vi "CRYO_DAQ_LSI218.vi"() -> ()   [LabVIEW 2017]
uses:
  USBData.lvclass
panel:
  in  "Stop Button":bool
  out "Cycle #":u32=16
  out "Time of Last Measurement":timestamp=timestamp(3679551576.02604 s since 1904-01-01)
  in  "wait (ms)":u32=1000
  in  "?":enum32{"CONFIG", "MEASUREMENT"}(tab)
  in  "USBSettings":T1(array[cluster])=[{"Label"="GXS450", "FileFormat"="%2.2f", "Physical CH"="Dev2/ai0", "ConversionType"={"Type"=enum."CC-10_LOG", "ConversionParameters"=[0.5, 9.0, 0.0, 1.0]}, "VoltageLimits"=[0.0, 10.0]}, {"Label"="Vacuum insluation", "FileFormat"="%2.2f", "Physical CH"="Dev2/ai1", "ConversionType"={"Type"=enum."CC-10_LOG", "ConversionParameters"=[0.5, 9.0, 0.0, 1.0]}, "VoltageLimits"=[0.0, 10.0]}, {"Label"="LeakDet_EXP", "FileFormat"="%2.2f", "Physical CH"="Dev2/ai2", "ConversionType"={"Type"=enum."LeakDet_EXP", "ConversionParameters"=[0.0, 1.0, 0.0, 1.0]}, "VoltageLimits"=[0.0, 10.0]}, {"Label"="LeakDet_Mantissa", "FileFormat"="%2.2f", "Physical CH"="Dev2/ai3", "ConversionType"={"Type"=enum."LeakDet_Mantissa", "ConversionParameters"=[0.0, 1.0, 0.0, 1.0]}, "VoltageLimits"=[0.0, 10.0]}]
  in  "RUN identifier":string="TEST"
  in  "Base Path":path=path "C:/LabVIEW/DATA/TestData/TestSeries"
  in  "Activate":bool=TRUE
  out "error out":errorcluster
  in  "InstName":string="USB6210"
  out "Status":T2(ring)=enum."Waiting"
  out "LeakRate":dbl=7.949318547575629e-10 format="%_3e"
  in  "Take Screenshot! 1":bool
  in  "Screenshot suffix 1":string="Graph1"
  in  "log/linear 2":bool
  in  "Plot in \nGraph2?":bool[](array[boolean])=[FALSE, TRUE, FALSE, FALSE, FALSE, FALSE]
  out "Graph 2":T3(graph)=[{"TimeArray"=[timestamp(3679551561.0226974 s since 1904-01-01), timestamp(3679551562.0229497 s since 1904-01-01), timestamp(3679551563.0239553 s since 1904-01-01), timestamp(3679551564.0244727 s since 1904-01-01), timestamp(3679551565.024744 s since 1904-01-01), timestamp(3679551566.0242834 s since 1904-01-01), timestamp(3679551567.023924 s since 1904-01-01), timestamp(3679551568.024467 s since 1904-01-01), timestamp(3679551569.024043 s since 1904-01-01), timestamp(3679551570.0247025 s since 1904-01-01), timestamp(3679551571.0251784 s since 1904-01-01), timestamp(3679551572.0251746 s since 1904-01-01), timestamp(3679551573.025196 s since 1904-01-01), timestamp(3679551574.0254583 s since 1904-01-01), timestamp(3679551575.0254254 s since 1904-01-01), timestamp(3679551576.02604 s since 1904-01-01)], "DataArray"=[3.4902207452388727, 3.4638947532560844, 3.5156819024300687, 3.5199434523425164, 3.4649439699863525, 3.5231430024807957, 3.502928189093684, 3.321102357963601, 3.4754536341457976, 3.499746997665005, 3.457606122570315, 3.4221855814628745, 3.3963727716400287, 3.480720413902356, 3.3861022462255765, 3.481774727194126]}, {"TimeArray"=[timestamp(3679551561.0226974 s since 1904-01-01), timestamp(3679551562.0229497 s since 1904-01-01), timestamp(3679551563.0239553 s since 1904-01-01), timestamp(3679551564.0244727 s since 1904-01-01), timestamp(3679551565.024744 s since 1904-01-01), timestamp(3679551566.0242834 s since 1904-01-01), timestamp(3679551567.023924 s since 1904-01-01), timestamp(3679551568.024467 s since 1904-01-01), timestamp(3679551569.024043 s since 1904-01-01), timestamp(3679551570.0247025 s since 1904-01-01), timestamp(3679551571.0251784 s since 1904-01-01), timestamp(3679551572.0251746 s since 1904-01-01), timestamp(3679551573.025196 s since 1904-01-01), timestamp(3679551574.0254583 s since 1904-01-01), timestamp(3679551575.0254254 s since 1904-01-01), timestamp(3679551576.02604 s since 1904-01-01)], "DataArray"=[16.893569884053267, 16.84758570488826, 16.90380557222128, 17.058087839454764, 17.423578167487687, 16.96021304914397, 17.146138727176098, 16.65480637969455, 16.924295644905385, 16.811906818948223, 17.016808777962343, 16.399538673319455, 16.604442643673547, 17.068423249776693, 16.133518383250625, 16.77630349203043]}, {"TimeArray"=[timestamp(3679551561.0226974 s since 1904-01-01), timestamp(3679551562.0229497 s since 1904-01-01), timestamp(3679551563.0239553 s since 1904-01-01), timestamp(3679551564.0244727 s since 1904-01-01), timestamp(3679551565.024744 s since 1904-01-01), timestamp(3679551566.0242834 s since 1904-01-01), timestamp(3679551567.023924 s since 1904-01-01), timestamp(3679551568.024467 s since 1904-01-01), timestamp(3679551569.024043 s since 1904-01-01), timestamp(3679551570.0247025 s since 1904-01-01), timestamp(3679551571.0251784 s since 1904-01-01), timestamp(3679551572.0251746 s since 1904-01-01), timestamp(3679551573.025196 s since 1904-01-01), timestamp(3679551574.0254583 s since 1904-01-01), timestamp(3679551575.0254254 s since 1904-01-01), timestamp(3679551576.02604 s since 1904-01-01)], "DataArray"=[-9.0, -9.0, -10.0, -10.0, -10.0, -10.0, -10.0, -10.0, -10.0, -10.0, -10.0, -10.0, -10.0, -10.0, -10.0, -10.0]}, {"TimeArray"=[timestamp(3679551561.0226974 s since 1904-01-01), timestamp(3679551562.0229497 s since 1904-01-01), timestamp(3679551563.0239553 s since 1904-01-01), timestamp(3679551564.0244727 s since 1904-01-01), timestamp(3679551565.024744 s since 1904-01-01), timestamp(3679551566.0242834 s since 1904-01-01), timestamp(3679551567.023924 s since 1904-01-01), timestamp(3679551568.024467 s since 1904-01-01), timestamp(3679551569.024043 s since 1904-01-01), timestamp(3679551570.0247025 s since 1904-01-01), timestamp(3679551571.0251784 s since 1904-01-01), timestamp(3679551572.0251746 s since 1904-01-01), timestamp(3679551573.025196 s since 1904-01-01), timestamp(3679551574.0254583 s since 1904-01-01), timestamp(3679551575.0254254 s since 1904-01-01), timestamp(3679551576.02604 s since 1904-01-01)], "DataArray"=[7.501070328753177, 7.449840163061198, 7.459770527105006, 7.50409547075007, 7.558285032992953, 7.615433997687735, 7.671070409569175, 7.724733918683316, 7.7683355340248115, 7.807728256473996, 7.842517497580663, 7.869020460156193, 7.896772947485954, 7.916567970959052, 7.934718892015823, 7.949318547575629]}, {"TimeArray"=[timestamp(3679551561.0226974 s since 1904-01-01), timestamp(3679551562.0229497 s since 1904-01-01), timestamp(3679551563.0239553 s since 1904-01-01), timestamp(3679551564.0244727 s since 1904-01-01), timestamp(3679551565.024744 s since 1904-01-01), timestamp(3679551566.0242834 s since 1904-01-01), timestamp(3679551567.023924 s since 1904-01-01), timestamp(3679551568.024467 s since 1904-01-01), timestamp(3679551569.024043 s since 1904-01-01), timestamp(3679551570.0247025 s since 1904-01-01), timestamp(3679551571.0251784 s since 1904-01-01), timestamp(3679551572.0251746 s since 1904-01-01), timestamp(3679551573.025196 s since 1904-01-01), timestamp(3679551574.0254583 s since 1904-01-01), timestamp(3679551575.0254254 s since 1904-01-01), timestamp(3679551576.02604 s since 1904-01-01)], "DataArray"=[7.501070328753178e-09, 7.4498401630611985e-09, 7.459770527105006e-10, 7.504095470750071e-10, 7.558285032992953e-10, 7.615433997687735e-10, 7.671070409569176e-10, 7.724733918683316e-10, 7.768335534024812e-10, 7.807728256473996e-10, 7.842517497580663e-10, 7.869020460156193e-10, 7.896772947485955e-10, 7.916567970959053e-10, 7.934718892015823e-10, 7.949318547575629e-10]}] caption="XY Graph"
  out "Graph 1":T4(graph)=[{"TimeArray"=[timestamp(3679551561.0226974 s since 1904-01-01), timestamp(3679551562.0229497 s since 1904-01-01), timestamp(3679551563.0239553 s since 1904-01-01), timestamp(3679551564.0244727 s since 1904-01-01), timestamp(3679551565.024744 s since 1904-01-01), timestamp(3679551566.0242834 s since 1904-01-01), timestamp(3679551567.023924 s since 1904-01-01), timestamp(3679551568.024467 s since 1904-01-01), timestamp(3679551569.024043 s since 1904-01-01), timestamp(3679551570.0247025 s since 1904-01-01), timestamp(3679551571.0251784 s since 1904-01-01), timestamp(3679551572.0251746 s since 1904-01-01), timestamp(3679551573.025196 s since 1904-01-01), timestamp(3679551574.0254583 s since 1904-01-01), timestamp(3679551575.0254254 s since 1904-01-01), timestamp(3679551576.02604 s since 1904-01-01)], "LDArray"=[3.4902207452388727, 3.4638947532560844, 3.5156819024300687, 3.5199434523425164, 3.4649439699863525, 3.5231430024807957, 3.502928189093684, 3.321102357963601, 3.4754536341457976, 3.499746997665005, 3.457606122570315, 3.4221855814628745, 3.3963727716400287, 3.480720413902356, 3.3861022462255765, 3.481774727194126]}, {"TimeArray"=[timestamp(3679551561.0226974 s since 1904-01-01), timestamp(3679551562.0229497 s since 1904-01-01), timestamp(3679551563.0239553 s since 1904-01-01), timestamp(3679551564.0244727 s since 1904-01-01), timestamp(3679551565.024744 s since 1904-01-01), timestamp(3679551566.0242834 s since 1904-01-01), timestamp(3679551567.023924 s since 1904-01-01), timestamp(3679551568.024467 s since 1904-01-01), timestamp(3679551569.024043 s since 1904-01-01), timestamp(3679551570.0247025 s since 1904-01-01), timestamp(3679551571.0251784 s since 1904-01-01), timestamp(3679551572.0251746 s since 1904-01-01), timestamp(3679551573.025196 s since 1904-01-01), timestamp(3679551574.0254583 s since 1904-01-01), timestamp(3679551575.0254254 s since 1904-01-01), timestamp(3679551576.02604 s since 1904-01-01)], "LDArray"=[16.893569884053267, 16.84758570488826, 16.90380557222128, 17.058087839454764, 17.423578167487687, 16.96021304914397, 17.146138727176098, 16.65480637969455, 16.924295644905385, 16.811906818948223, 17.016808777962343, 16.399538673319455, 16.604442643673547, 17.068423249776693, 16.133518383250625, 16.77630349203043]}, {"TimeArray"=[timestamp(3679551561.0226974 s since 1904-01-01), timestamp(3679551562.0229497 s since 1904-01-01), timestamp(3679551563.0239553 s since 1904-01-01), timestamp(3679551564.0244727 s since 1904-01-01), timestamp(3679551565.024744 s since 1904-01-01), timestamp(3679551566.0242834 s since 1904-01-01), timestamp(3679551567.023924 s since 1904-01-01), timestamp(3679551568.024467 s since 1904-01-01), timestamp(3679551569.024043 s since 1904-01-01), timestamp(3679551570.0247025 s since 1904-01-01), timestamp(3679551571.0251784 s since 1904-01-01), timestamp(3679551572.0251746 s since 1904-01-01), timestamp(3679551573.025196 s since 1904-01-01), timestamp(3679551574.0254583 s since 1904-01-01), timestamp(3679551575.0254254 s since 1904-01-01), timestamp(3679551576.02604 s since 1904-01-01)], "LDArray"=[-9.0, -9.0, -10.0, -10.0, -10.0, -10.0, -10.0, -10.0, -10.0, -10.0, -10.0, -10.0, -10.0, -10.0, -10.0, -10.0]}, {"TimeArray"=[timestamp(3679551561.0226974 s since 1904-01-01), timestamp(3679551562.0229497 s since 1904-01-01), timestamp(3679551563.0239553 s since 1904-01-01), timestamp(3679551564.0244727 s since 1904-01-01), timestamp(3679551565.024744 s since 1904-01-01), timestamp(3679551566.0242834 s since 1904-01-01), timestamp(3679551567.023924 s since 1904-01-01), timestamp(3679551568.024467 s since 1904-01-01), timestamp(3679551569.024043 s since 1904-01-01), timestamp(3679551570.0247025 s since 1904-01-01), timestamp(3679551571.0251784 s since 1904-01-01), timestamp(3679551572.0251746 s since 1904-01-01), timestamp(3679551573.025196 s since 1904-01-01), timestamp(3679551574.0254583 s since 1904-01-01), timestamp(3679551575.0254254 s since 1904-01-01), timestamp(3679551576.02604 s since 1904-01-01)], "LDArray"=[7.501070328753177, 7.449840163061198, 7.459770527105006, 7.50409547075007, 7.558285032992953, 7.615433997687735, 7.671070409569175, 7.724733918683316, 7.7683355340248115, 7.807728256473996, 7.842517497580663, 7.869020460156193, 7.896772947485954, 7.916567970959052, 7.934718892015823, 7.949318547575629]}, {"TimeArray"=[timestamp(3679551561.0226974 s since 1904-01-01), timestamp(3679551562.0229497 s since 1904-01-01), timestamp(3679551563.0239553 s since 1904-01-01), timestamp(3679551564.0244727 s since 1904-01-01), timestamp(3679551565.024744 s since 1904-01-01), timestamp(3679551566.0242834 s since 1904-01-01), timestamp(3679551567.023924 s since 1904-01-01), timestamp(3679551568.024467 s since 1904-01-01), timestamp(3679551569.024043 s since 1904-01-01), timestamp(3679551570.0247025 s since 1904-01-01), timestamp(3679551571.0251784 s since 1904-01-01), timestamp(3679551572.0251746 s since 1904-01-01), timestamp(3679551573.025196 s since 1904-01-01), timestamp(3679551574.0254583 s since 1904-01-01), timestamp(3679551575.0254254 s since 1904-01-01), timestamp(3679551576.02604 s since 1904-01-01)], "LDArray"=[7.501070328753178e-09, 7.4498401630611985e-09, 7.459770527105006e-10, 7.504095470750071e-10, 7.558285032992953e-10, 7.615433997687735e-10, 7.671070409569176e-10, 7.724733918683316e-10, 7.768335534024812e-10, 7.807728256473996e-10, 7.842517497580663e-10, 7.869020460156193e-10, 7.896772947485955e-10, 7.916567970959053e-10, 7.934718892015823e-10, 7.949318547575629e-10]}] caption="XY Graph"
  out "LastData":dbl[](array[numeric])=[3.481774727194126, 16.77630349203043, -10.0, 7.949318547575629, 7.949318547575629e-10]
  out "AllSeries":string[](array[string])=["GXS450", "Vacuum inslation", "LeakDet_EXP", "LeakDet_Mantissa", "LaekDet_FULL"]
  in  "Plot in \nGraph1?":bool[](array[boolean])=[TRUE, FALSE, FALSE, FALSE, FALSE, FALSE]
  in  "log/linear 1":bool=TRUE
  in  "Take Screenshot! 2":bool
  in  "Screenshot suffix 2":string="Graph2"
  # "GLOBAL STATUS/CONTROL"
  # "USB6210 Settings"
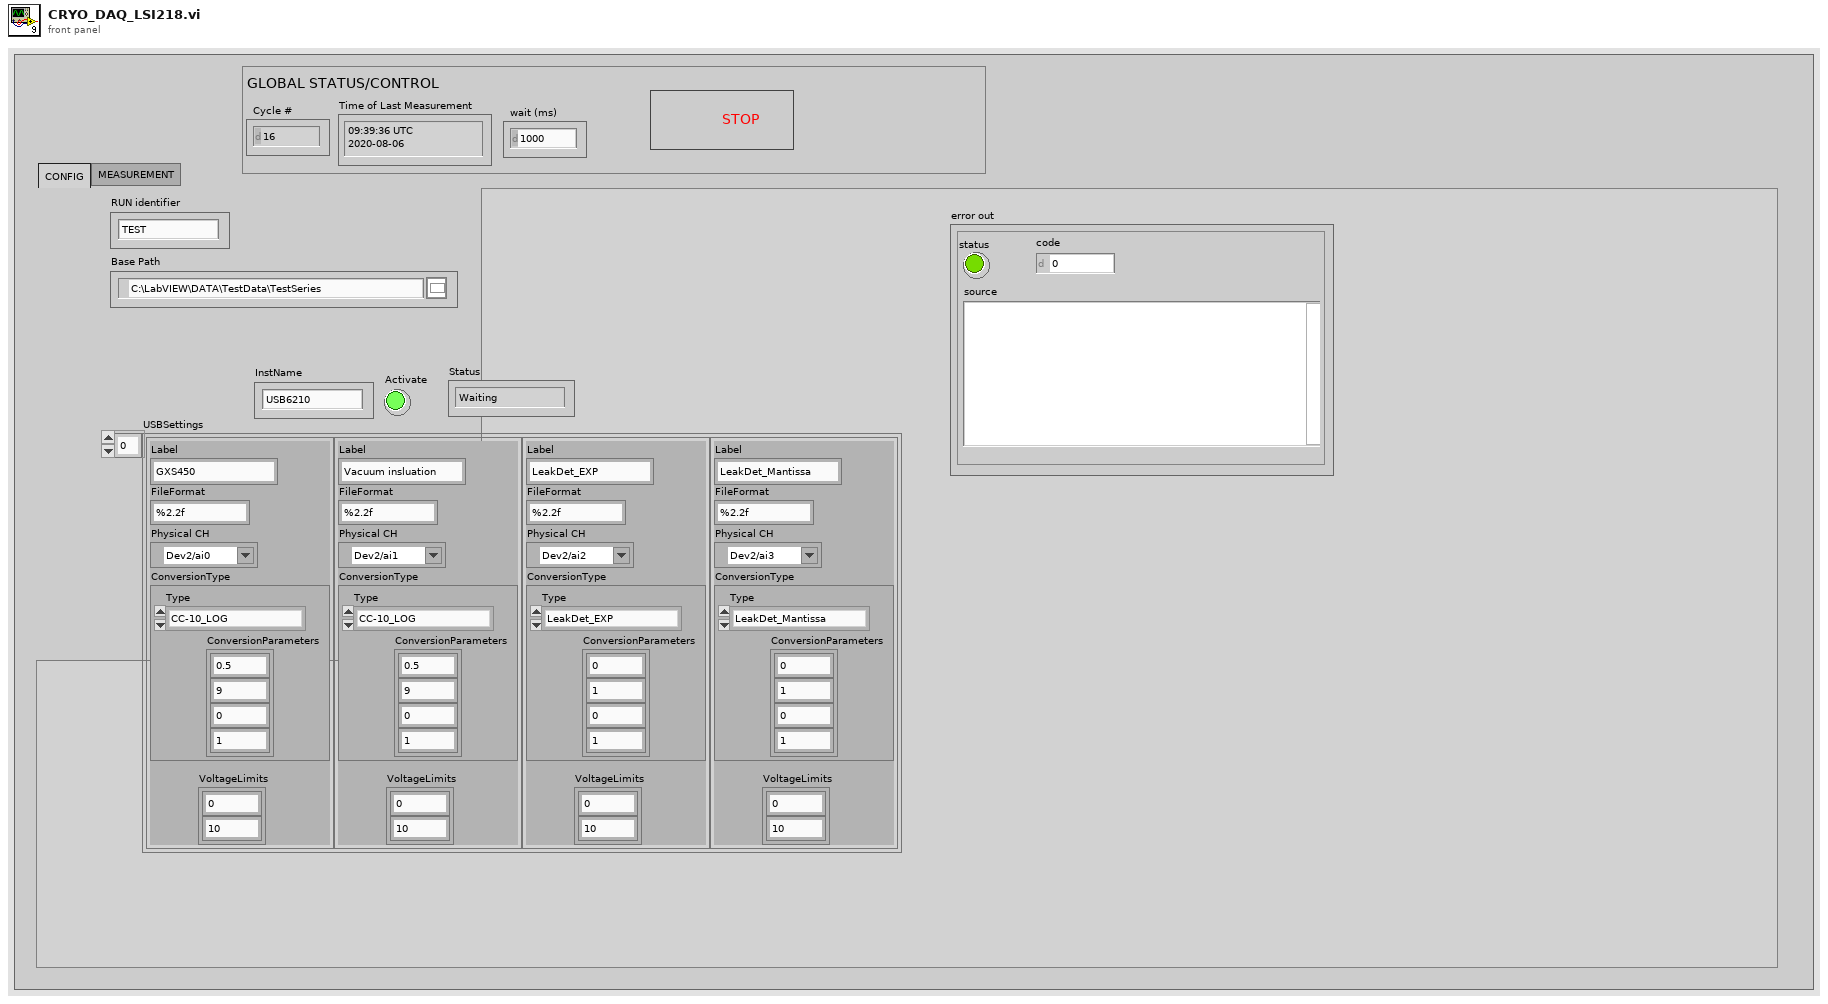
[diagram p1: front panel]
types:
  T1 = cluster{"Label":string, "FileFormat":string, "Physical CH":tag, "ConversionType":cluster{"Type":enum16{"Raw", "SimpleProp", "CC-10_COMBINED", "CC-10_LOG", "LeakDet_EXP", "LeakDet_Mantissa", "Baratron"}, "ConversionParameters":dbl[]}, "VoltageLimits":dbl[]}[]
  T2 = enum16{"Intialized", "Waiting", "Measuring", "Terminated"}
  T3 = cluster{"TimeArray":timestamp[], "DataArray":dbl[]}[]
  T4 = cluster{"TimeArray":timestamp[], "LDArray":dbl[]}[]
  T5 = cluster{"TimeArray":timestamp[], "DataArrayConv":dbl[]}[]
  T6 = cluster{"IndexArray":i64[], "TimeArray":timestamp[], "DataArrayRaw":dbl[][], "DataArrayConv":dbl[][], "LDArray":dbl[]}
  T7 = cluster{"InstName":string, "Active?":bool, "Status":enum16{"Intialized", "Waiting", "Measuring", "Terminated"}, "Labels":string[], "LabelLD":string, "FileFormat":string[], "FileFormatLD":string, "ReadLeakDet?":bool}
  T8 = cluster{"TimeArray":timestamp[], "DataArrayConv":dbl[]}
  T9 = cluster{"TimeArray":timestamp[], "LDArray":dbl[]}
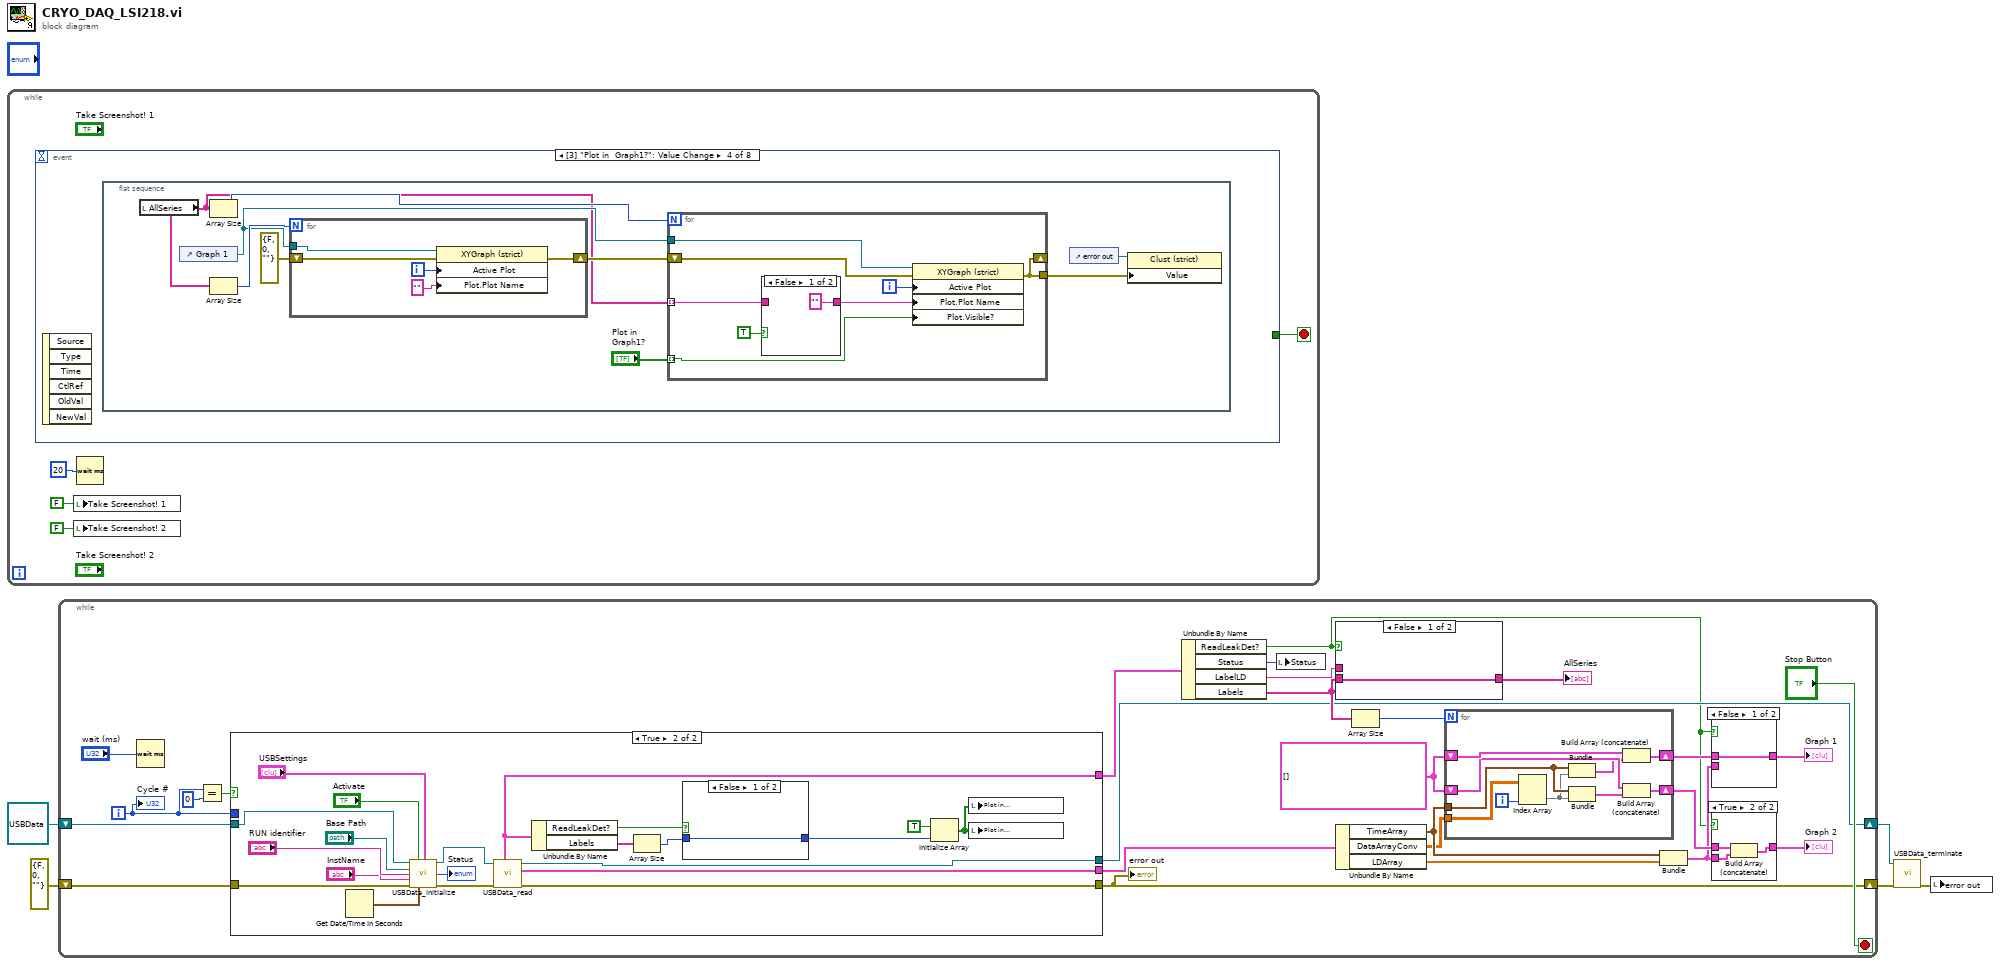
[diagram p0: block diagram]
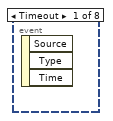
[diagram p2: hidden frame]
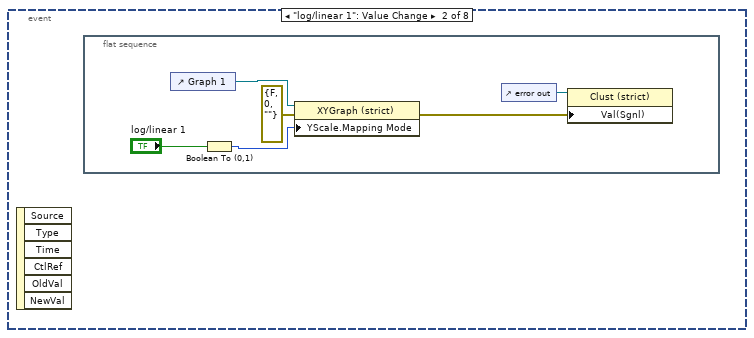
[diagram p3: hidden frame]
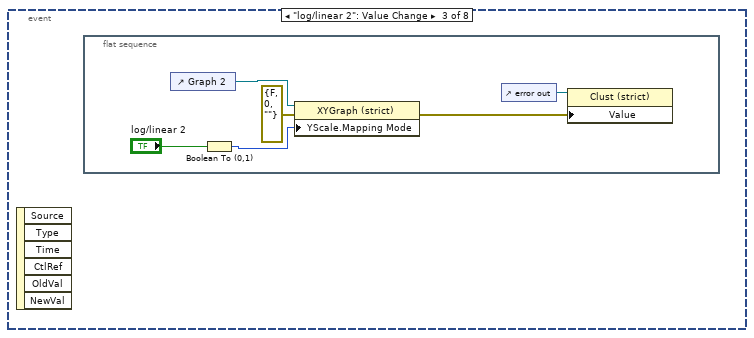
[diagram p4: hidden frame]
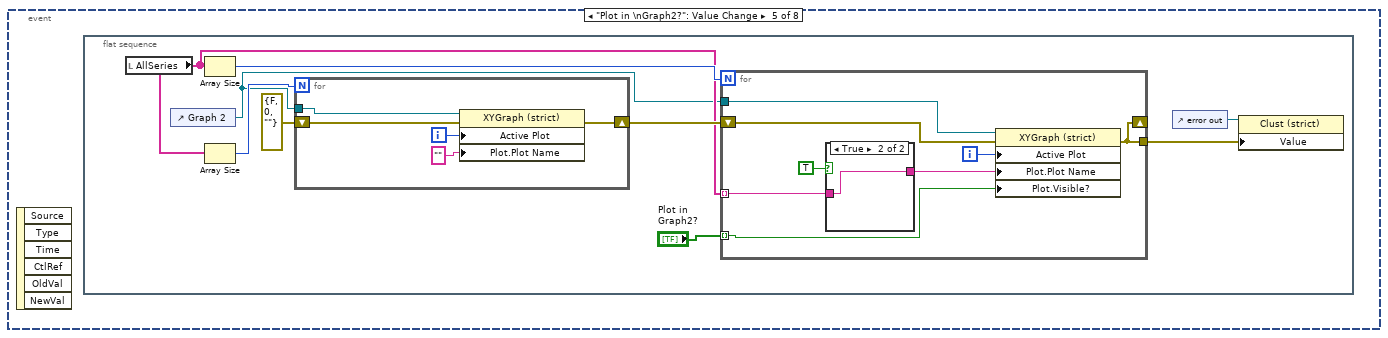
[diagram p6: hidden frame]
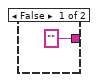
[diagram p7: hidden frame]
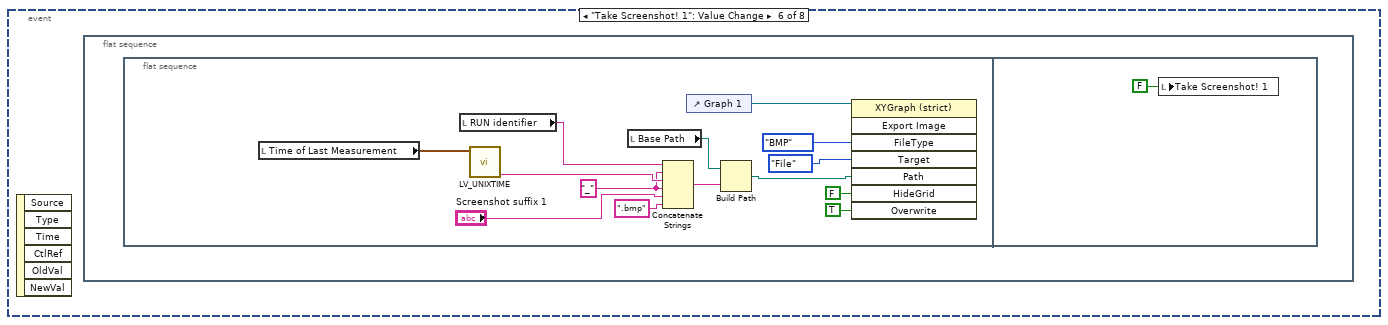
[diagram p8: hidden frame]
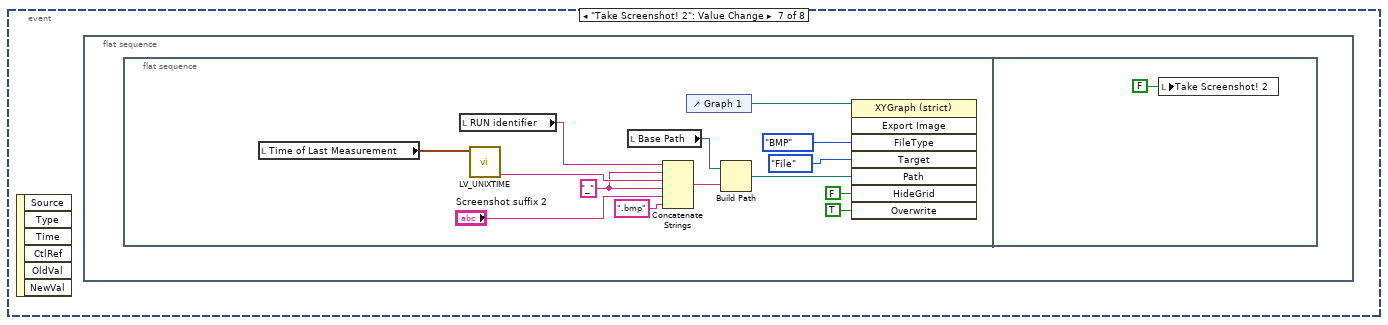
[diagram p9: hidden frame]
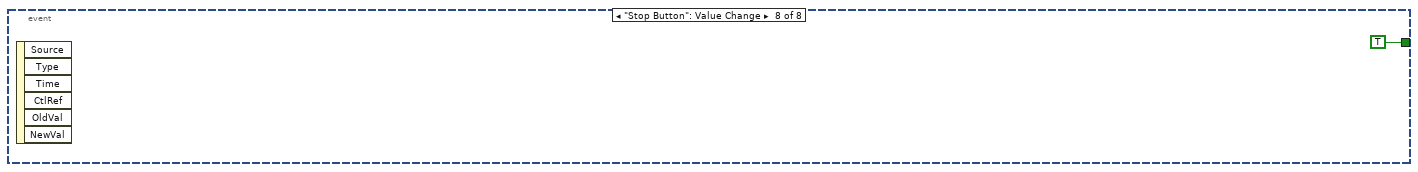
[diagram p10: hidden frame]
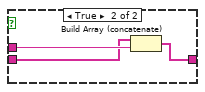
[diagram p11: hidden frame]
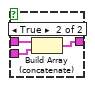
[diagram p13: hidden frame]
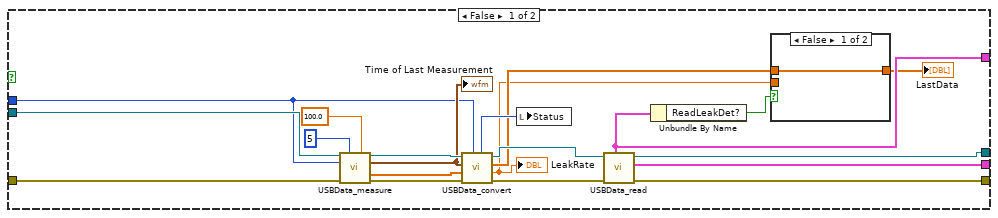
[diagram p14: hidden frame]
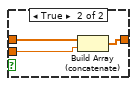
[diagram p15: hidden frame]
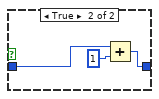
[diagram p16: hidden frame]
diagram:
  n1 = while {
    stop <- w8 stop-if-true
    n2 = event shown="[3] \"Plot in  Graph1?\": Value Change" {
      selector: _ -> [_ _ _ _ _ _ _ _]
      dyn-events: _ -> [_ _ _ _ _ _ _ _]
      timeout: _ -> [_ _ _ _ _ _ _ _]
      tunnel: [_ _ _ _ _ _ _ TRUE] -> w8
      event Timeout {
        n3 = event-data() -> ()  [unwired: 1 in, 3 out]
      }
      event "log/linear 1": Value Change {
        n4 = event-data() -> ()  [unwired: 1 in, 6 out]
        n5 = flat-sequence {
          frame #0 {
            n6 = control-ref of="Graph 1"() -> (w13:refnum<vi>)
            n7 = Boolean To (0,1)(Boolean="log/linear 1") -> (0, 1=w14:i16)
            n8 = property class="XYGraph (strict)"(reference=w13, error in=errorcluster {"status"=FALSE, "code"=0, "source"=""} ("error in (no error)"), "YScale.Mapping Mode"=w14) -> (error out=w11:errorcluster)  [unwired: 1 out]
            n9 = control-ref of="error out"() -> (w12:refnum<vi>)
            n10 = property class="Clust (strict)"(reference=w12, "Val(Sgnl)"=w11) -> ()  [unwired: 1 in, 2 out]
          }
        }
      }
      event "log/linear 2": Value Change {
        n11 = event-data() -> ()  [unwired: 1 in, 6 out]
        n12 = flat-sequence {
          frame #0 {
            n13 = control-ref of="Graph 2"() -> (w17:refnum<vi>)
            n14 = Boolean To (0,1)(Boolean="log/linear 2") -> (0, 1=w20:i16)
            n15 = property class="XYGraph (strict)"(reference=w17, error in=errorcluster {"status"=FALSE, "code"=0, "source"=""} ("error in (no error)"), "YScale.Mapping Mode"=w20) -> (error out=w19:errorcluster)  [unwired: 1 out]
            n16 = control-ref of="error out"() -> (w16:refnum<vi>)
            n17 = property class="Clust (strict)"(reference=w16, "Value"=w19) -> ()  [unwired: 1 in, 2 out]
          }
        }
      }
      event "Plot in \nGraph1?": Value Change {
        n18 = event-data() -> ()  [unwired: 1 in, 6 out]
        n19 = flat-sequence {
          frame #0 {
            n20 = local read "AllSeries"() -> (w23:string[])
            n21 = control-ref of="Graph 1"() -> (w27:refnum<vi>)
            n22 = Array Size(array=w23) -> (size(s)=w28:i32)
            n23 = Array Size(array=w23) -> (size(s)=w29:i32)
            n24 = for {
              N: w29 -> [_]
              tunnel: w27 -> [w43]
              shift-right: [w41] -> w25
              shift-left: errorcluster {"status"=FALSE, "code"=0, "source"=""} ("error in (no error)") -> [w42]
              i -> [w45]
              n25 = property class="XYGraph (strict)"(reference=w43, error in=w42, "Active Plot"=w45, "Plot.Plot Name"="") -> (error out=w41:errorcluster)  [unwired: 1 out]
            }
            n26 = for {
              N: w28 -> [_]
              tunnel: w27 -> [w37]
              shift-right: [w35] -> _
              shift-left: w25 -> [w36]
              tunnel: [w35] -> w24
              tunnel: "Plot in \nGraph1?" -> [w32] mode=indexing
              tunnel: w23 -> [w33] mode=indexing
              i -> [w38]
              n27 = case shown="False" TRUE {
                tunnel: ["" ("Plot.Plot Name") w40] -> w34
                tunnel: w33 -> [_ w40]
                frame False {
                }
                frame True {
                }
              }
              n28 = property class="XYGraph (strict)"(reference=w37, error in=w36, "Active Plot"=w38, "Plot.Plot Name"=w34, "Plot.Visible?"=w32) -> (error out=w35:errorcluster)  [unwired: 1 out]
            }
            n29 = control-ref of="error out"() -> (w30:refnum<vi>)
            n30 = property class="Clust (strict)"(reference=w30, "Value"=w24) -> ()  [unwired: 1 in, 2 out]
          }
        }
      }
      event "Plot in \nGraph2?": Value Change {
        n31 = event-data() -> ()  [unwired: 1 in, 6 out]
        n32 = flat-sequence {
          frame #0 {
            n33 = local read "AllSeries"() -> (w48:string[])
            n34 = control-ref of="Graph 2"() -> (w46:refnum<vi>)
            n35 = Array Size(array=w48) -> (size(s)=w52:i32)
            n36 = Array Size(array=w48) -> (size(s)=w53:i32)
            n37 = for {
              N: w53 -> [_]
              shift-right: [w66] -> w50
              shift-left: errorcluster {"status"=FALSE, "code"=0, "source"=""} ("error in (no error)") -> [w67]
              tunnel: w46 -> [w65]
              i -> [w69]
              n38 = property class="XYGraph (strict)"(reference=w65, error in=w67, "Active Plot"=w69, "Plot.Plot Name"="") -> (error out=w66:errorcluster)  [unwired: 1 out]
            }
            n39 = for {
              N: w52 -> [_]
              shift-right: [w60] -> _
              shift-left: w50 -> [w61]
              tunnel: [w60] -> w49
              tunnel: w48 -> [w58] mode=indexing
              tunnel: "Plot in \nGraph2?" -> [w57] mode=indexing
              tunnel: w46 -> [w56]
              i -> [w62]
              n40 = case shown="True" TRUE {
                tunnel: ["" ("Plot.Plot Name") w64] -> w59
                tunnel: w58 -> [_ w64]
                frame False {
                }
                frame True {
                }
              }
              n41 = property class="XYGraph (strict)"(reference=w56, error in=w61, "Active Plot"=w62, "Plot.Plot Name"=w59, "Plot.Visible?"=w57) -> (error out=w60:errorcluster)  [unwired: 1 out]
            }
            n42 = control-ref of="error out"() -> (w54:refnum<vi>)
            n43 = property class="Clust (strict)"(reference=w54, "Value"=w49) -> ()  [unwired: 1 in, 2 out]
          }
        }
      }
      event "Take Screenshot! 1": Value Change {
        n44 = event-data() -> ()  [unwired: 1 in, 6 out]
        n45 = flat-sequence {
          frame #0 {
            n46 = flat-sequence {
              frame #0 {
                w72 = "_" ("string")
                n47 = local read "Time of Last Measurement"() -> (w74:timestamp)
                n48 = local read "RUN identifier"() -> (w77:string)
                n49 = call "LV_UNIXTIME.vi"("current time"=w74) -> ("date/time string"=w73:string)  [unwired: 9 in, 1 out]
                n50 = local read "Base Path"() -> (w78:path)
                n51 = Concatenate Strings(w77, w72, w73, w72, "Screenshot suffix 1", ".bmp" ("string")) -> (w83:string)
                n52 = control-ref of="Graph 1"() -> (w75:refnum<vi>)
                n53 = Build Path(base path=w78, name or relative path=w83) -> (appended path=w82:path)
                n54 = invoke on="Invoke Node" class="XYGraph (strict)" method="Export Image"(reference=w75, "FileType"=enum32{"BMP", "EPS", "EMF", "PICT"}."BMP" ("File Type"), "Target"=enum32{"File", "Clipboard"}."File", "Path"=w82, "HideGrid"=FALSE ("Hide Grid"), "Overwrite"=TRUE ("Always Overwrite")) -> ()  [unwired: 2 in, 8 out]
              }
              frame #1 {
                n55 = local write "Take Screenshot! 1"(FALSE ("Take Screenshot! 1")) -> ()
              }
            }
          }
        }
      }
      event "Take Screenshot! 2": Value Change {
        n56 = event-data() -> ()  [unwired: 1 in, 6 out]
        n57 = flat-sequence {
          frame #0 {
            n58 = flat-sequence {
              frame #0 {
                w87 = "_" ("string")
                n59 = local read "Time of Last Measurement"() -> (w89:timestamp)
                n60 = local read "RUN identifier"() -> (w92:string)
                n61 = call "LV_UNIXTIME.vi"("current time"=w89) -> ("date/time string"=w88:string)  [unwired: 9 in, 1 out]
                n62 = local read "Base Path"() -> (w93:path)
                n63 = Concatenate Strings(w92, w87, w88, w87, "Screenshot suffix 2", ".bmp" ("string")) -> (w98:string)
                n64 = control-ref of="Graph 1"() -> (w90:refnum<vi>)
                n65 = Build Path(base path=w93, name or relative path=w98) -> (appended path=w97:path)
                n66 = invoke on="Invoke Node" class="XYGraph (strict)" method="Export Image"(reference=w90, "FileType"=enum32{"BMP", "EPS", "EMF", "PICT"}."BMP" ("File Type"), "Target"=enum32{"File", "Clipboard"}."File", "Path"=w97, "HideGrid"=FALSE ("Hide Grid"), "Overwrite"=TRUE ("Always Overwrite")) -> ()  [unwired: 2 in, 8 out]
              }
              frame #1 {
                n67 = local write "Take Screenshot! 2"(FALSE ("Take Screenshot! 1")) -> ()
              }
            }
          }
        }
      }
      event "Stop Button": Value Change {
        n68 = event-data() -> ()  [unwired: 1 in, 6 out]
      }
    }
    n69 = local write "Take Screenshot! 1"(FALSE ("Take Screenshot! 1")) -> ()
    n70 = local write "Take Screenshot! 2"(FALSE ("Take Screenshot! 1")) -> ()
    n71 = Wait (ms)(milliseconds to wait=u32 20) -> ()  [unwired: 1 out]
  }
  n72 = while {
    shift-right: [w103] -> w2
    shift-left: refnum<class "USBData.lvclass"> refnum ("USBData.lvclass") -> [w123]
    shift-right: [w102] -> w1
    shift-left: errorcluster {"status"=FALSE, "code"=0, "source"=""} ("error in (no error)") -> [w122]
    i -> [w109]
    stop <- "Stop Button" stop-if-true
    w112 = T5 [] ("appended array")
    n73 = Wait (ms)(milliseconds to wait="wait (ms)") -> ()  [unwired: 1 out]
    n74 = Equal?(x=w109, y=0) -> (x = y?=w124:bool)
    n75 = case shown="True" w124 {
      tunnel: w123 -> [w168 w193]
      tunnel: w122 -> [w162 w187]
      tunnel: w109 -> [w159 _]
      tunnel: [w157 w182] -> w102
      tunnel: [w154 w181] -> w105
      tunnel: [w155 w180] -> w103
      tunnel: [w151 w173] -> w104
      frame False {
        n76 = call-dynamic "USBData_measure.vi"("USBData in"=w168, "DAQ sample #"=i64 5, "DAQ timeout"=100.0 ("DAQ timeout (def: 100)"), "MeasurementIndex"=w159, "error in (no error)"=w162) -> ("USBData out"=w167:refnum<class "USBData.lvclass">, "TimeMeasuremeent"=w164:timestamp, "LastDataAcquired"=w160:dbl[], "error out"=w163:errorcluster)  [unwired: 4 in, 3 out]
        "Time of Last Measurement" <- w164
        n77 = call-dynamic "USBData_convert.vi"("MeasurementIndex"=w159, "error in (no error)"=w163, "LastDataAcquired"=w160, "TimeMeasuremeent"=w164, "USBData in"=w167) -> ("error out"=w158:errorcluster, "LeakDet_FULL"=w152:dbl, "LastDataConverted"=w153:dbl[], "USBData out"=w156:refnum<class "USBData.lvclass">, "Status"=w161:T2)  [unwired: 2 in]
        "LeakRate" <- w152
        n78 = local write "Status"(w161) -> ()
        n79 = call "USBData_read.vi"("error in (no error)"=w158, "USBData in"=w156) -> ("error out"=w157:errorcluster, "Data"=w154:T6, "USBData out"=w155:refnum<class "USBData.lvclass">, "Basic"=w151:T7)  [unwired: 3 in, 1 out]
        n80 = Unbundle By Name(w151) -> ("ReadLeakDet?"=w150:bool)
        n81 = case shown="False" w150 {
          tunnel: w153 -> [w169 w172]
          tunnel: w152 -> [_ w171]
          tunnel: [w169 w170] -> w149
          frame False {
          }
          frame True {
            n82 = Build Array (concatenate)(w172, w171) -> (w170:dbl[])
          }
        }
        "LastData" <- w149
      }
      frame True {
        n83 = Get Date/Time In Seconds() -> (seconds since 1Jan1904=w188:timestamp)
        n84 = call-dynamic "USBData_initialize.vi"("USBData in"=w193, "Activate?"="Activate", "SeriesSetting"="USBSettings", "BasePath"="Base Path", "RunName"="RUN identifier", "InstName"="InstName", "error in (no error)"=w187, "RUN start time"=w188) -> ("USBData out"=w183:refnum<class "USBData.lvclass">, "Status"=→"Status":T2, "error out"=w184:errorcluster)  [unwired: 3 in, 2 out]
        n85 = call "USBData_read.vi"("error in (no error)"=w184, "USBData in"=w183) -> ("error out"=w182:errorcluster, "Data"=w181:T6, "USBData out"=w180:refnum<class "USBData.lvclass">, "Basic"=w173:T7)  [unwired: 3 in, 1 out]
        n86 = Unbundle By Name(w173) -> ("ReadLeakDet?"=w178:bool, "Labels"=w179:string[])
        n87 = Array Size(array=w179) -> (size(s)=w177:i32)
        n88 = case shown="False" w178 {
          tunnel: w177 -> [w194 w196]
          tunnel: [w194 w195] -> w175
          frame False {
          }
          frame True {
            n89 = Add(x=w196, y=1) -> (x+y=w195:i32)
          }
        }
        n90 = Initialize Array(TRUE ("Activate 2"), w175) -> (w174:bool[])
        n91 = local write "Plot in \nGraph2?"(w174) -> ()
        n92 = local write "Plot in \nGraph1?"(w174) -> ()
      }
    }
    "error out" <- w102
    n93 = Unbundle By Name(w104) -> ("ReadLeakDet?"=w101:bool, "Status"=w120:T2, "LabelLD"=w119:string, "Labels"=w106:string[])
    n94 = local write "Status"(w120) -> ()
    n95 = case shown="False" w101 {
      tunnel: w119 -> [_ w130]
      tunnel: [w127 w129] -> w107
      tunnel: w106 -> [w127 w128]
      frame False {
      }
      frame True {
        n96 = Build Array (concatenate)(w128, w130) -> (w129:string[])
      }
    }
    "AllSeries" <- w107
    n97 = Unbundle By Name(w105) -> ("TimeArray"=w121:timestamp[], "DataArrayConv"=w115:dbl[][], "LDArray"=w114:dbl[])
    n98 = Array Size(array=w106) -> (size(s)=w116:i32)
    n99 = for {
      N: w116 -> [_]
      tunnel: w115 -> [w144]
      tunnel: w121 -> [w148]
      shift-right: [w142] -> w118
      shift-left: w112 -> [w146]
      shift-right: [w139] -> w113
      shift-left: w112 -> [w147]
      i -> [w145]
      n100 = Index Array(array=w144, index (col)=w145) -> (element=w143:dbl[])  [unwired: 1 in]
      n101 = Bundle("TimeArray"=w148, "DataArrayConv"=w143) -> (w140:T8)  [unwired: 1 in]
      n102 = Bundle("TimeArray"=w148, "DataArrayConv"=w143) -> (w141:T8)  [unwired: 1 in]
      n103 = Build Array (concatenate)(w147, w140) -> (w139:T5)
      n104 = Build Array (concatenate)(w146, w141) -> (w142:T5)
    }
    n105 = Bundle("TimeArray"=w121, "LDArray"=w114) -> (w117:T9)  [unwired: 1 in]
    n106 = case shown="False" w101 {
      tunnel: w117 -> [_ w138]
      tunnel: [w135 w137] -> w111
      tunnel: w113 -> [w135 w136]
      frame False {
      }
      frame True {
        n107 = Build Array (concatenate)(w136, w138) -> (w137:T4)
      }
    }
    "Graph 1" <- w111
    n108 = case shown="True" w101 {
      tunnel: [w131 w134] -> w110
      tunnel: w118 -> [w131 w133]
      tunnel: w117 -> [_ w132]
      frame False {
      }
      frame True {
        n109 = Build Array (concatenate)(w133, w132) -> (w134:T4)
      }
    }
    "Graph 2" <- w110
    "Cycle #" <- w109
  }
  n110 = call-dynamic "USBData_terminate.vi"("error in (no error)"=w1, "USBData in"=w2) -> ("error out"=w3:errorcluster)  [unwired: 8 in, 1 out]
  n111 = local write "error out"(w3) -> ()
